vi "TDMS_Open - 1D - Copy.vi"(7 "Offset":bool, 10 "Input 2D":dbl[][](array[numeric]), 11 "Open":bool) -> (1 "Output 2D":dbl[][](array[numeric]), 3 "Freq_Sampling_SizeX_SizeY":dbl[](array[numeric]), 8 "Gate 2":dbl=15.0, 9 "Gate 1":dbl=5.0)   [LabVIEW 2012]
uses:
  <vilib>/Platform/NI_3dgraph.lvlib
panel:
  in  "Loop":i32
  in  "Step":dbl=5.0
  in  "milliseconds to wait":u32
  in  "3D Surface":refnum<k7>(container)
  in  "Samples per Channel":i32=1000 caption="Samples"
  in  "Rate":dbl=60000.0 caption="Sample Rate (Hz)" format="%0.0f"
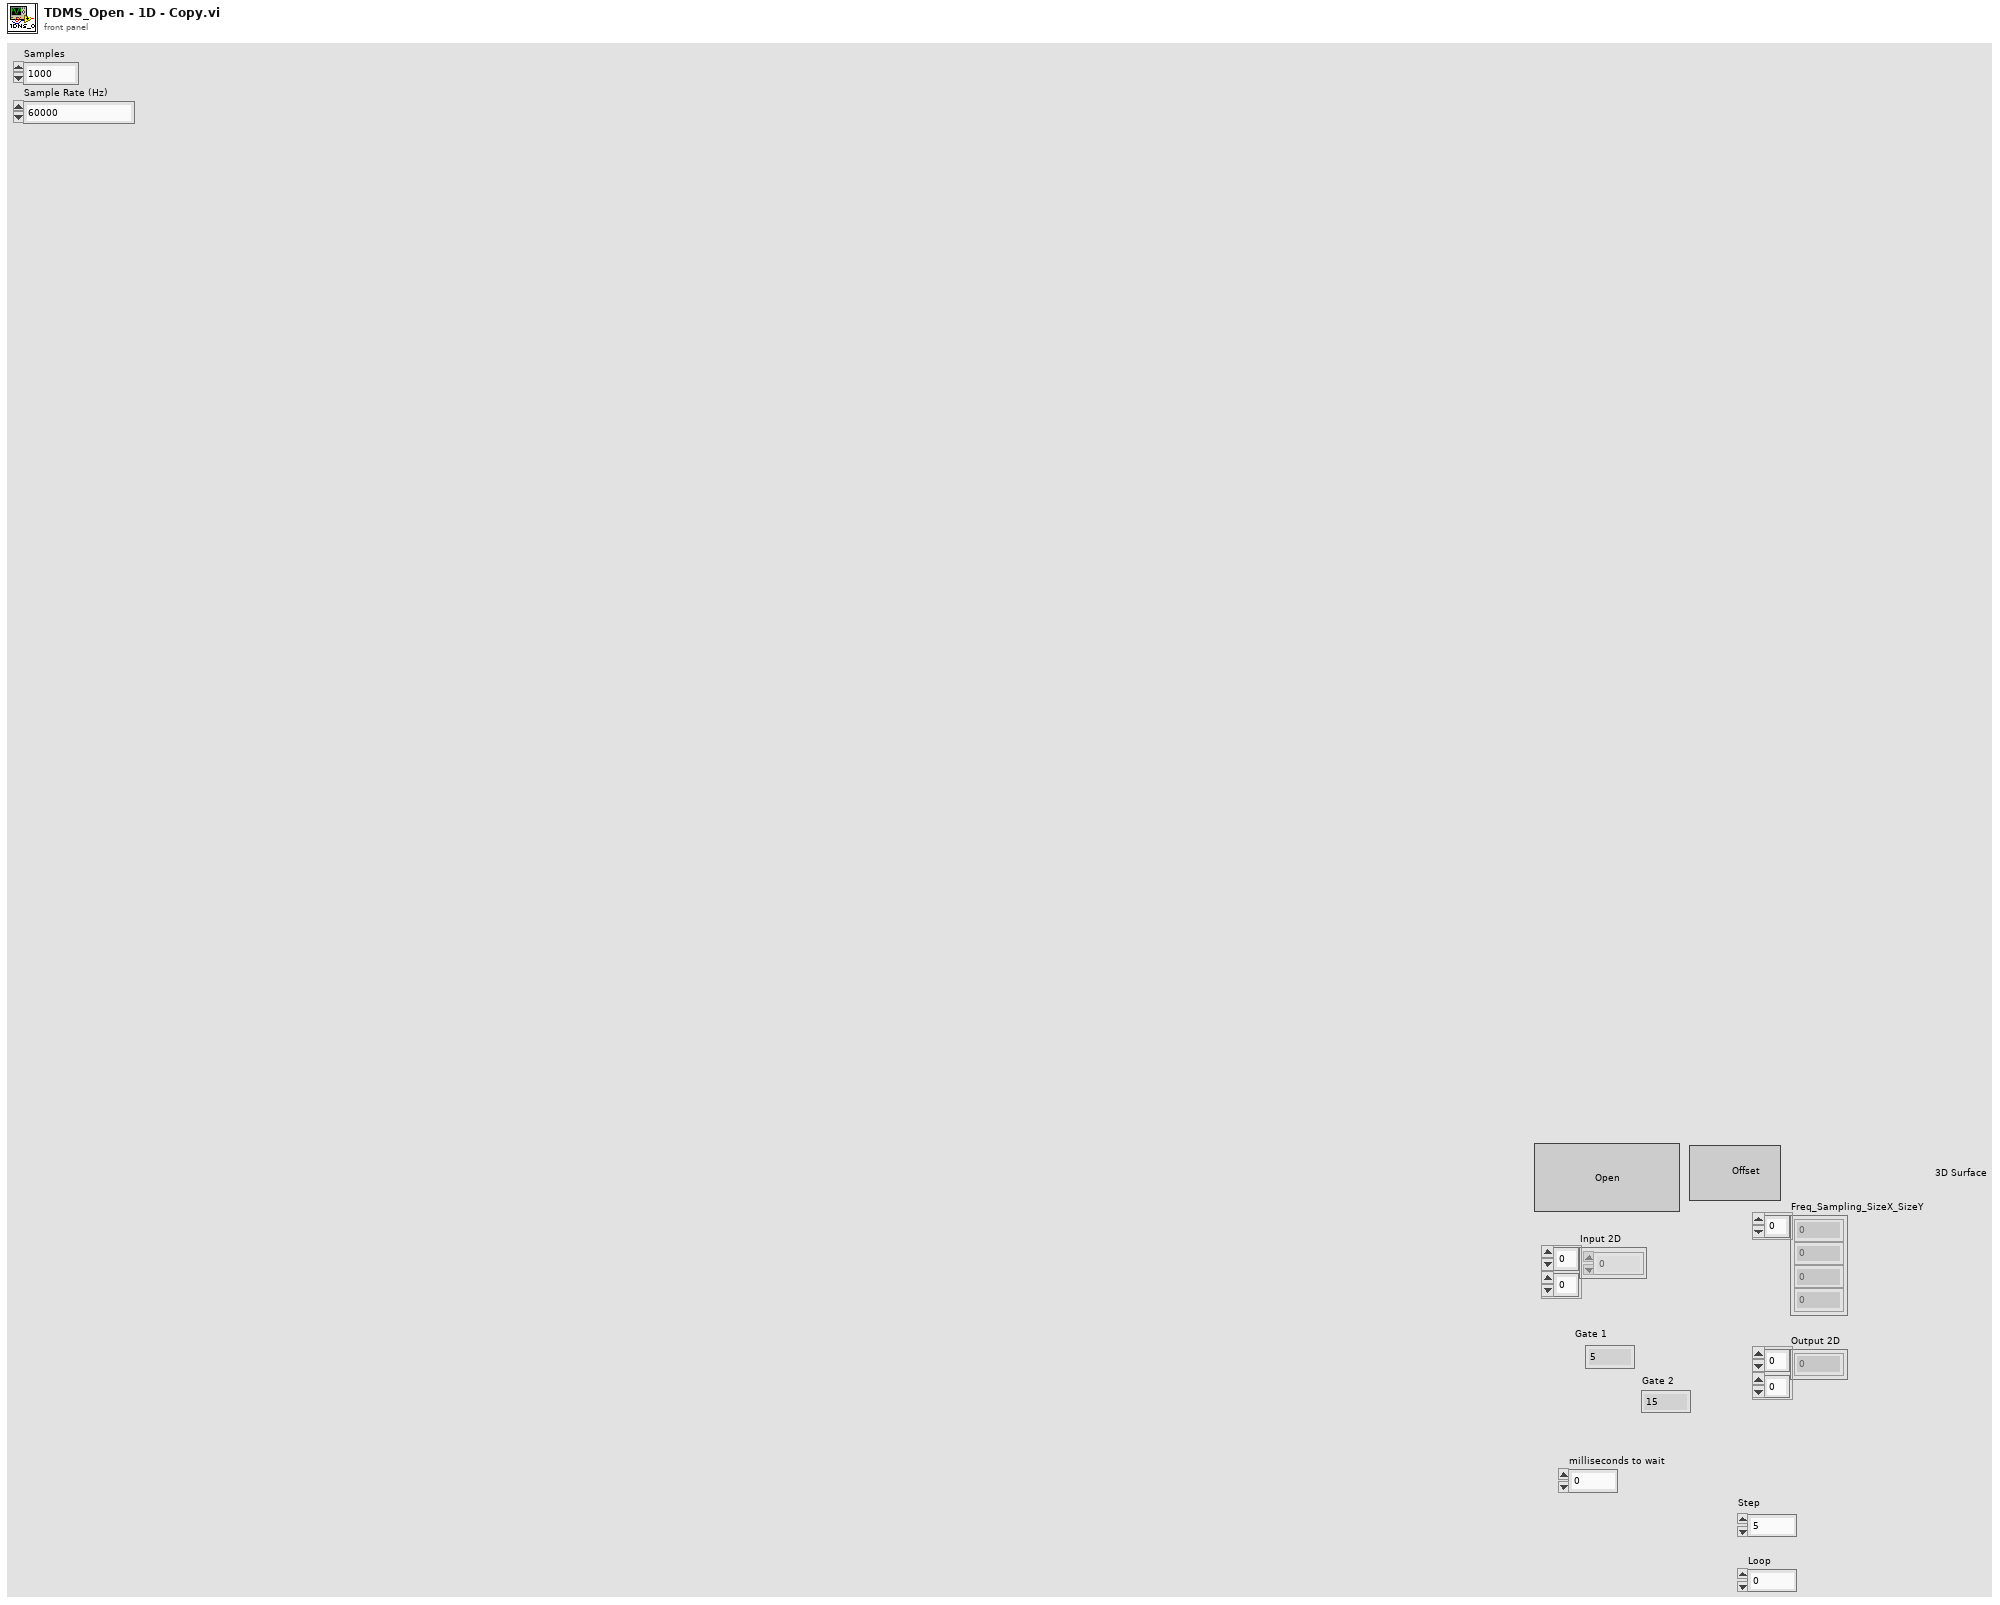
[diagram p1: front panel]
types:
  T1 = enum16{"open", "open or create", "create or replace", "create", "open (read-only)"}
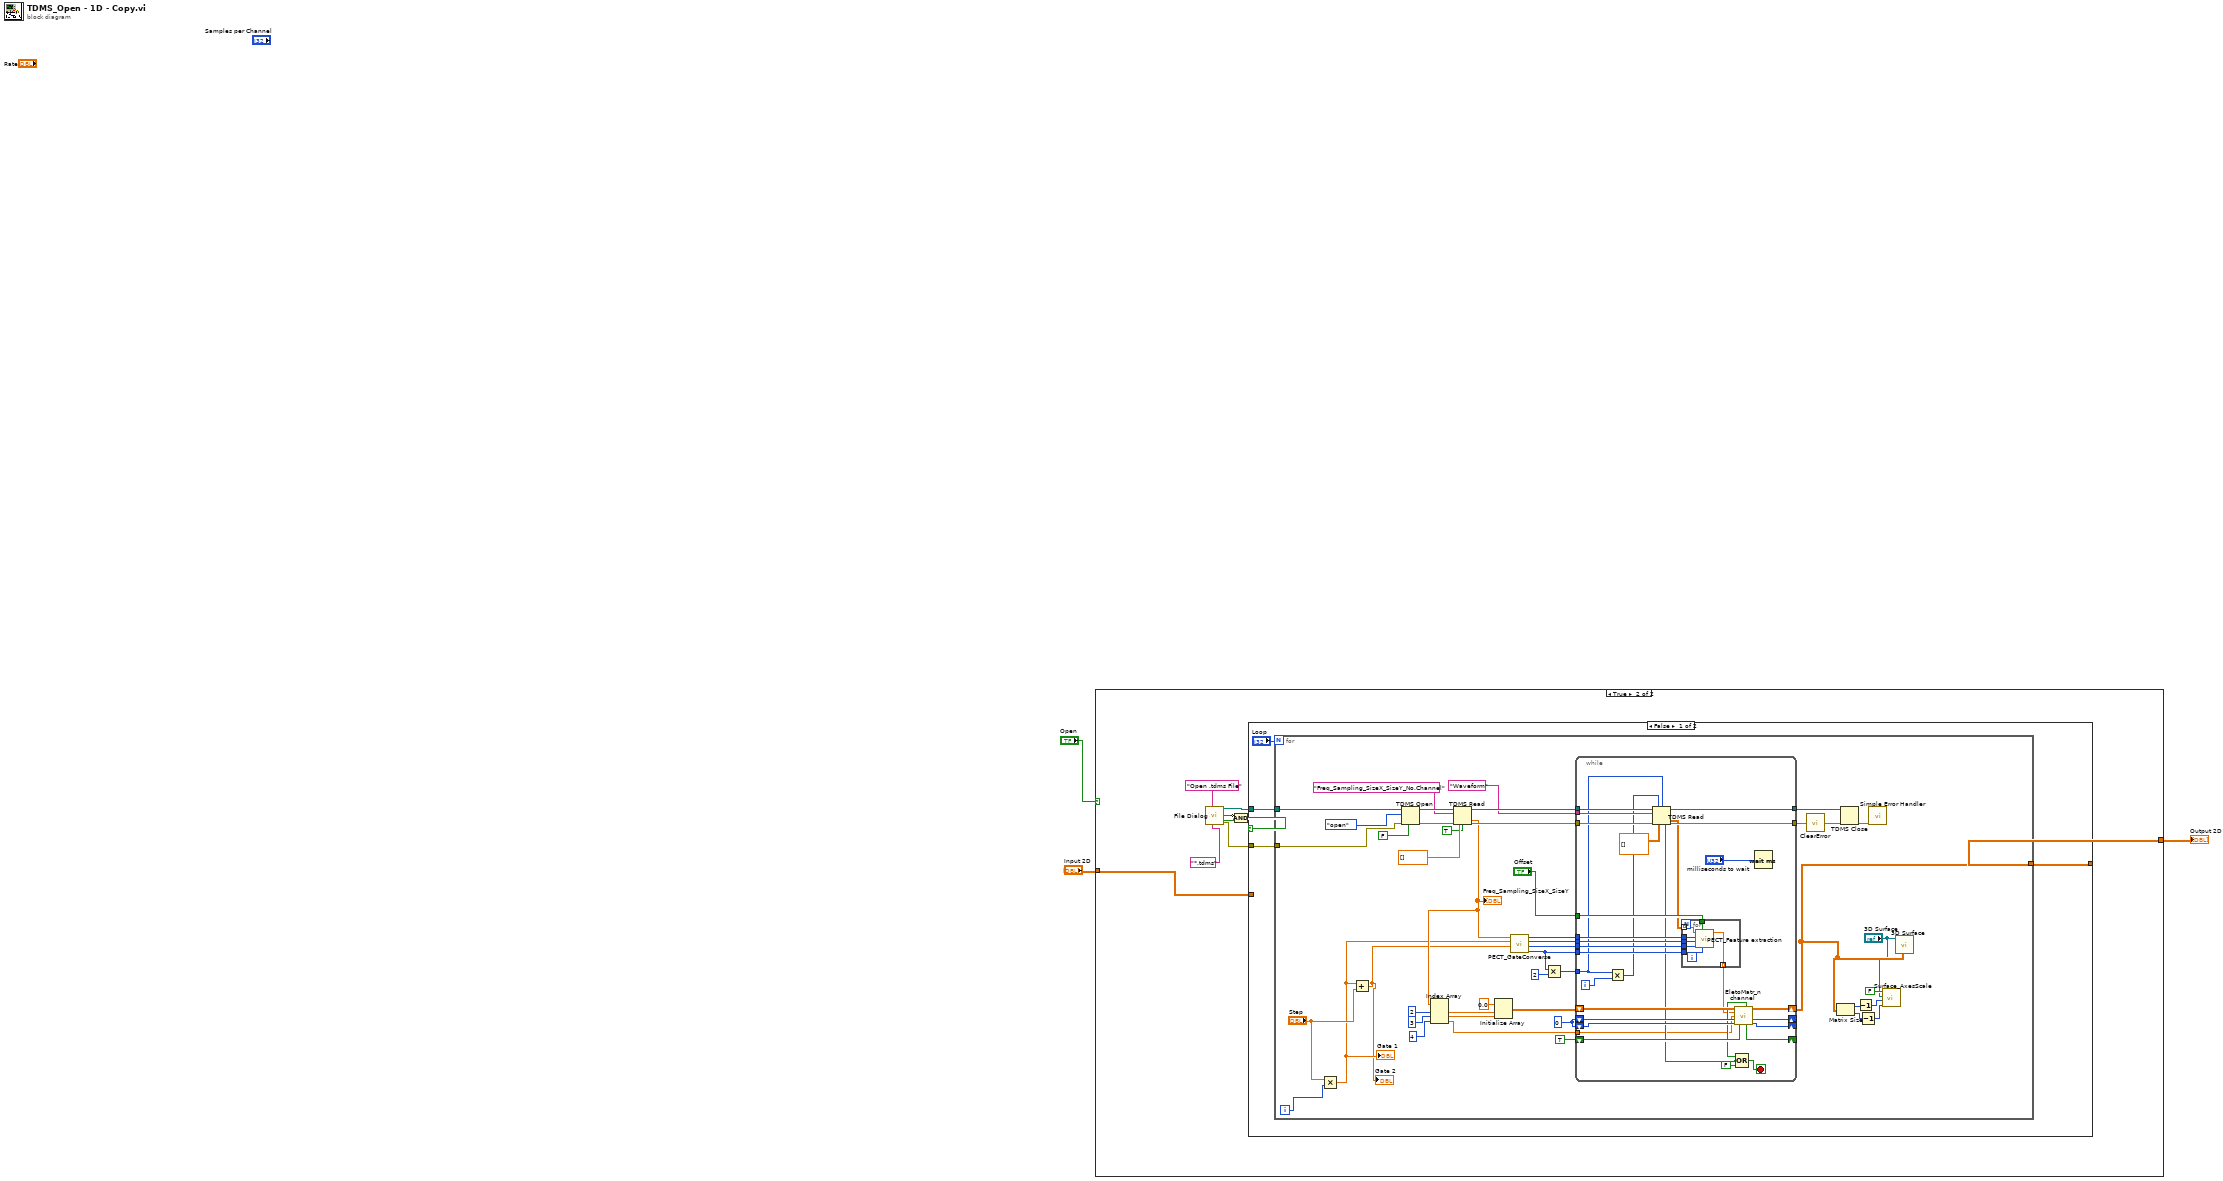
[diagram p0: block diagram]
diagram:
  n1 = case shown="True" "Open" {
    tunnel: [w4 w13] -> w1
    tunnel: "Input 2D" -> [w4 w12]
    frame False {
    }
    frame True {
      n2 = call "File Dialog"("prompt"="Open .tdms File" ("button label"), "pattern (all files)"="*.tdms") -> ("selected path"=w11:path, "exists"=w9:bool, "cancelled"=w8:bool, "error out"=w5:errorcluster)  [unwired: 10 in]
      n3 = Compound Arithmetic op=AND(invert w9, w8) -> (w7:bool)
      n4 = case shown="False" w7 {
        tunnel: w11 -> [w16 _]
        tunnel: [w15 w100] -> w13
        tunnel: w12 -> [_ w100]
        tunnel: w5 -> [w17 _]
        frame False {
          n5 = for {
            N: "Loop" -> [_]
            tunnel: w17 -> [w52]
            tunnel: w16 -> [w32]
            tunnel: [w22] -> w15
            i -> [w20]
            w41 = 0 ("Out Row")
            n6 = Multiply(x="Step", y=w20) -> (x*y=w19:dbl)
            "Gate 1" <- w19
            n7 = Add(x=w19, y="Step") -> (x+y=w18:dbl)
            "Gate 2" <- w18
            n8 = TDMS Open(6:FALSE ("disable buffering (T)"), 8:w52, 10:T1."open" ("operation"), 11:w32) -> (0:w58:errorcluster, 3:w62:refnum<k34>)  [unwired: 2 in]
            n9 = TDMS Read(0:w62, 5:"Freq_Sampling_SizeX_SizeY_No.Channel" ("group name in"), 11:w58, 12:dbl[] [] ("Array"), 13:TRUE ("return channels in file order? (F)")) -> (4:w36:refnum<k34>, 10:w31:dbl[], 15:w51:errorcluster)  [unwired: 3 in, 3 out]
            "Freq_Sampling_SizeX_SizeY" <- w31
            n10 = Index Array(array=w31, index #1=2 ("index"), index #2=3 ("index"), index #3=4 ("index")) -> (element #1=w43:dbl, element #2=w42:dbl, element #3=w29:dbl)
            n11 = Initialize Array(0.0 ("element"), w43, w42) -> (w44:dbl[][])
            n12 = call "PECT_GateConverse.vi"("Gate 2"=w18, "Gate 1"=w19, "Freq_Sampling_SizeX_SizeY"=w31) -> ("Length T/2"=w38:i32, "Length"=w48:i32, "Start 2"=w49:i32, "Start 1"=w50:i32)  [unwired: 5 in]
            n13 = Multiply(x=w38, y=2) -> (x*y=w37:i32)
            n14 = while {
              tunnel: [w92] -> w54
              tunnel: [w91] -> w53
              tunnel: "Waveform" ("group name in") -> [w72]
              tunnel: w36 -> [w89]
              tunnel: w51 -> [w88]
              tunnel: w50 -> [w87]
              tunnel: w49 -> [w86]
              tunnel: w48 -> [w85]
              shift-right: [w83] -> w22
              shift-left: w44 -> [w84]
              shift-right: [w80] -> _
              shift-left: w41 -> [w82]
              shift-right: [w79] -> _
              shift-left: w41 -> [w81]
              shift-right: [w77] -> _
              shift-left: TRUE ("Output Direction") -> [w78]
              tunnel: w37 -> [w70]
              tunnel: w38 -> [w76]
              tunnel: "Offset" -> [w73]
              tunnel: w29 -> [w64]
              i -> [w74]
              stop <- w67 stop-if-true
              n15 = Multiply(x=w70, y=w74) -> (x*y=w71:i32)
              n16 = TDMS Read(0:w89, 1:w71, 2:w70, 5:w72, 11:w88, 12:dbl[][] [] ("Array")) -> (4:w92:refnum<k34>, 10:w63:dbl[][], 14:w68:bool, 15:w91:errorcluster)  [unwired: 2 in, 2 out]
              n17 = for {
                tunnel: w87 -> [w99]
                tunnel: w86 -> [w98]
                tunnel: w85 -> [w97]
                tunnel: [w96] -> w65 mode=indexing
                tunnel: w76 -> [w95]
                tunnel: w73 -> [w94]
                tunnel: w63 -> [w93] mode=indexing
                n18 = call "PECT_Feature extraction.vi"("Length T/2"=w95, "Offset"=w94, "Length"=w97, "Start 2"=w98, "Start 1"=w99, "Pulse signal in"=w93) -> ("Feature extraction out"=w96:dbl)  [unwired: 5 in]
              }
              n19 = call "EletoMatr_n channel.vi"("Input Array X"=w84, "Input data"=w65, "No. channels"=w64, "In Row"=w82, "In Column"=w81, "Input Direction"=w78) -> ("Completed"=w69:bool, "Out Array X"=w83:dbl[][], "Out Row"=w80:i32, "Output Direction"=w77:bool, "Out Column"=w79:i32)  [unwired: 5 in]
              n20 = Compound Arithmetic op=OR(w69, w68, FALSE ("value")) -> (w67:bool)
              n21 = Wait (ms)(milliseconds to wait="milliseconds to wait") -> ()  [unwired: 1 out]
            }
            n22 = call <vilib>:"ClearError.vi"("error in (no error)"=w53) -> ("error out"=w56:errorcluster)
            n23 = Matrix Size(0:w22) -> (1:w25:i32, 2:w26:i32)
            n24 = TDMS Close(8:w56, 11:w54) -> (0:w55:errorcluster)  [unwired: 1 out]
            n25 = Decrement(x=w25) -> (x-1=w23:i32)
            n26 = Decrement(x=w26) -> (x-1=w27:i32)
            n27 = call <vilib>:"Simple Error Handler.vi"("error in (no error)"=w55) -> ()  [unwired: 1 in, 8 out]
            n28 = call "Surface_AxesScale.vi"("Y-axis Max"=w27, "X-axis max"=w23, "3D Surface"="3D Surface", "Auto Scale"=FALSE) -> ()  [unwired: 8 in]
            n29 = call <vilib>:"3D Surface.vi"("z matrix"=w22, "3D graph"="3D Surface") -> ()  [unwired: 8 in, 2 out]
          }
        }
        frame True {
        }
      }
    }
  }
  "Output 2D" <- w1
